vi "HEWH Water Cp.vi"(7 "Water Properties Reference":T1, 8 "Error In":errorcluster, 11 "Input Temperature (°F)":dbl format="%.4f") -> (0 "Error Out":errorcluster, 3 "Specific Heat (BTU/lbm*F)":dbl)   [LabVIEW 2019]
uses:
  Macros/UEF/Type Definitions/HEWH Water Properties.ctl
panel:
  out "Rounded Number":dbl
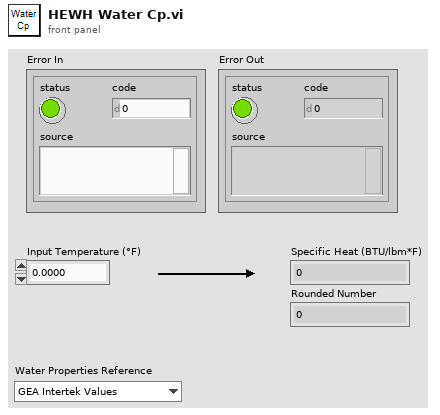
[diagram p1: front panel]
types:
  T1 = typedef "HEWH Water Properties.ctl" = enum16{"GEA Intertek Values", "CSA Values", "ANSI Values"}
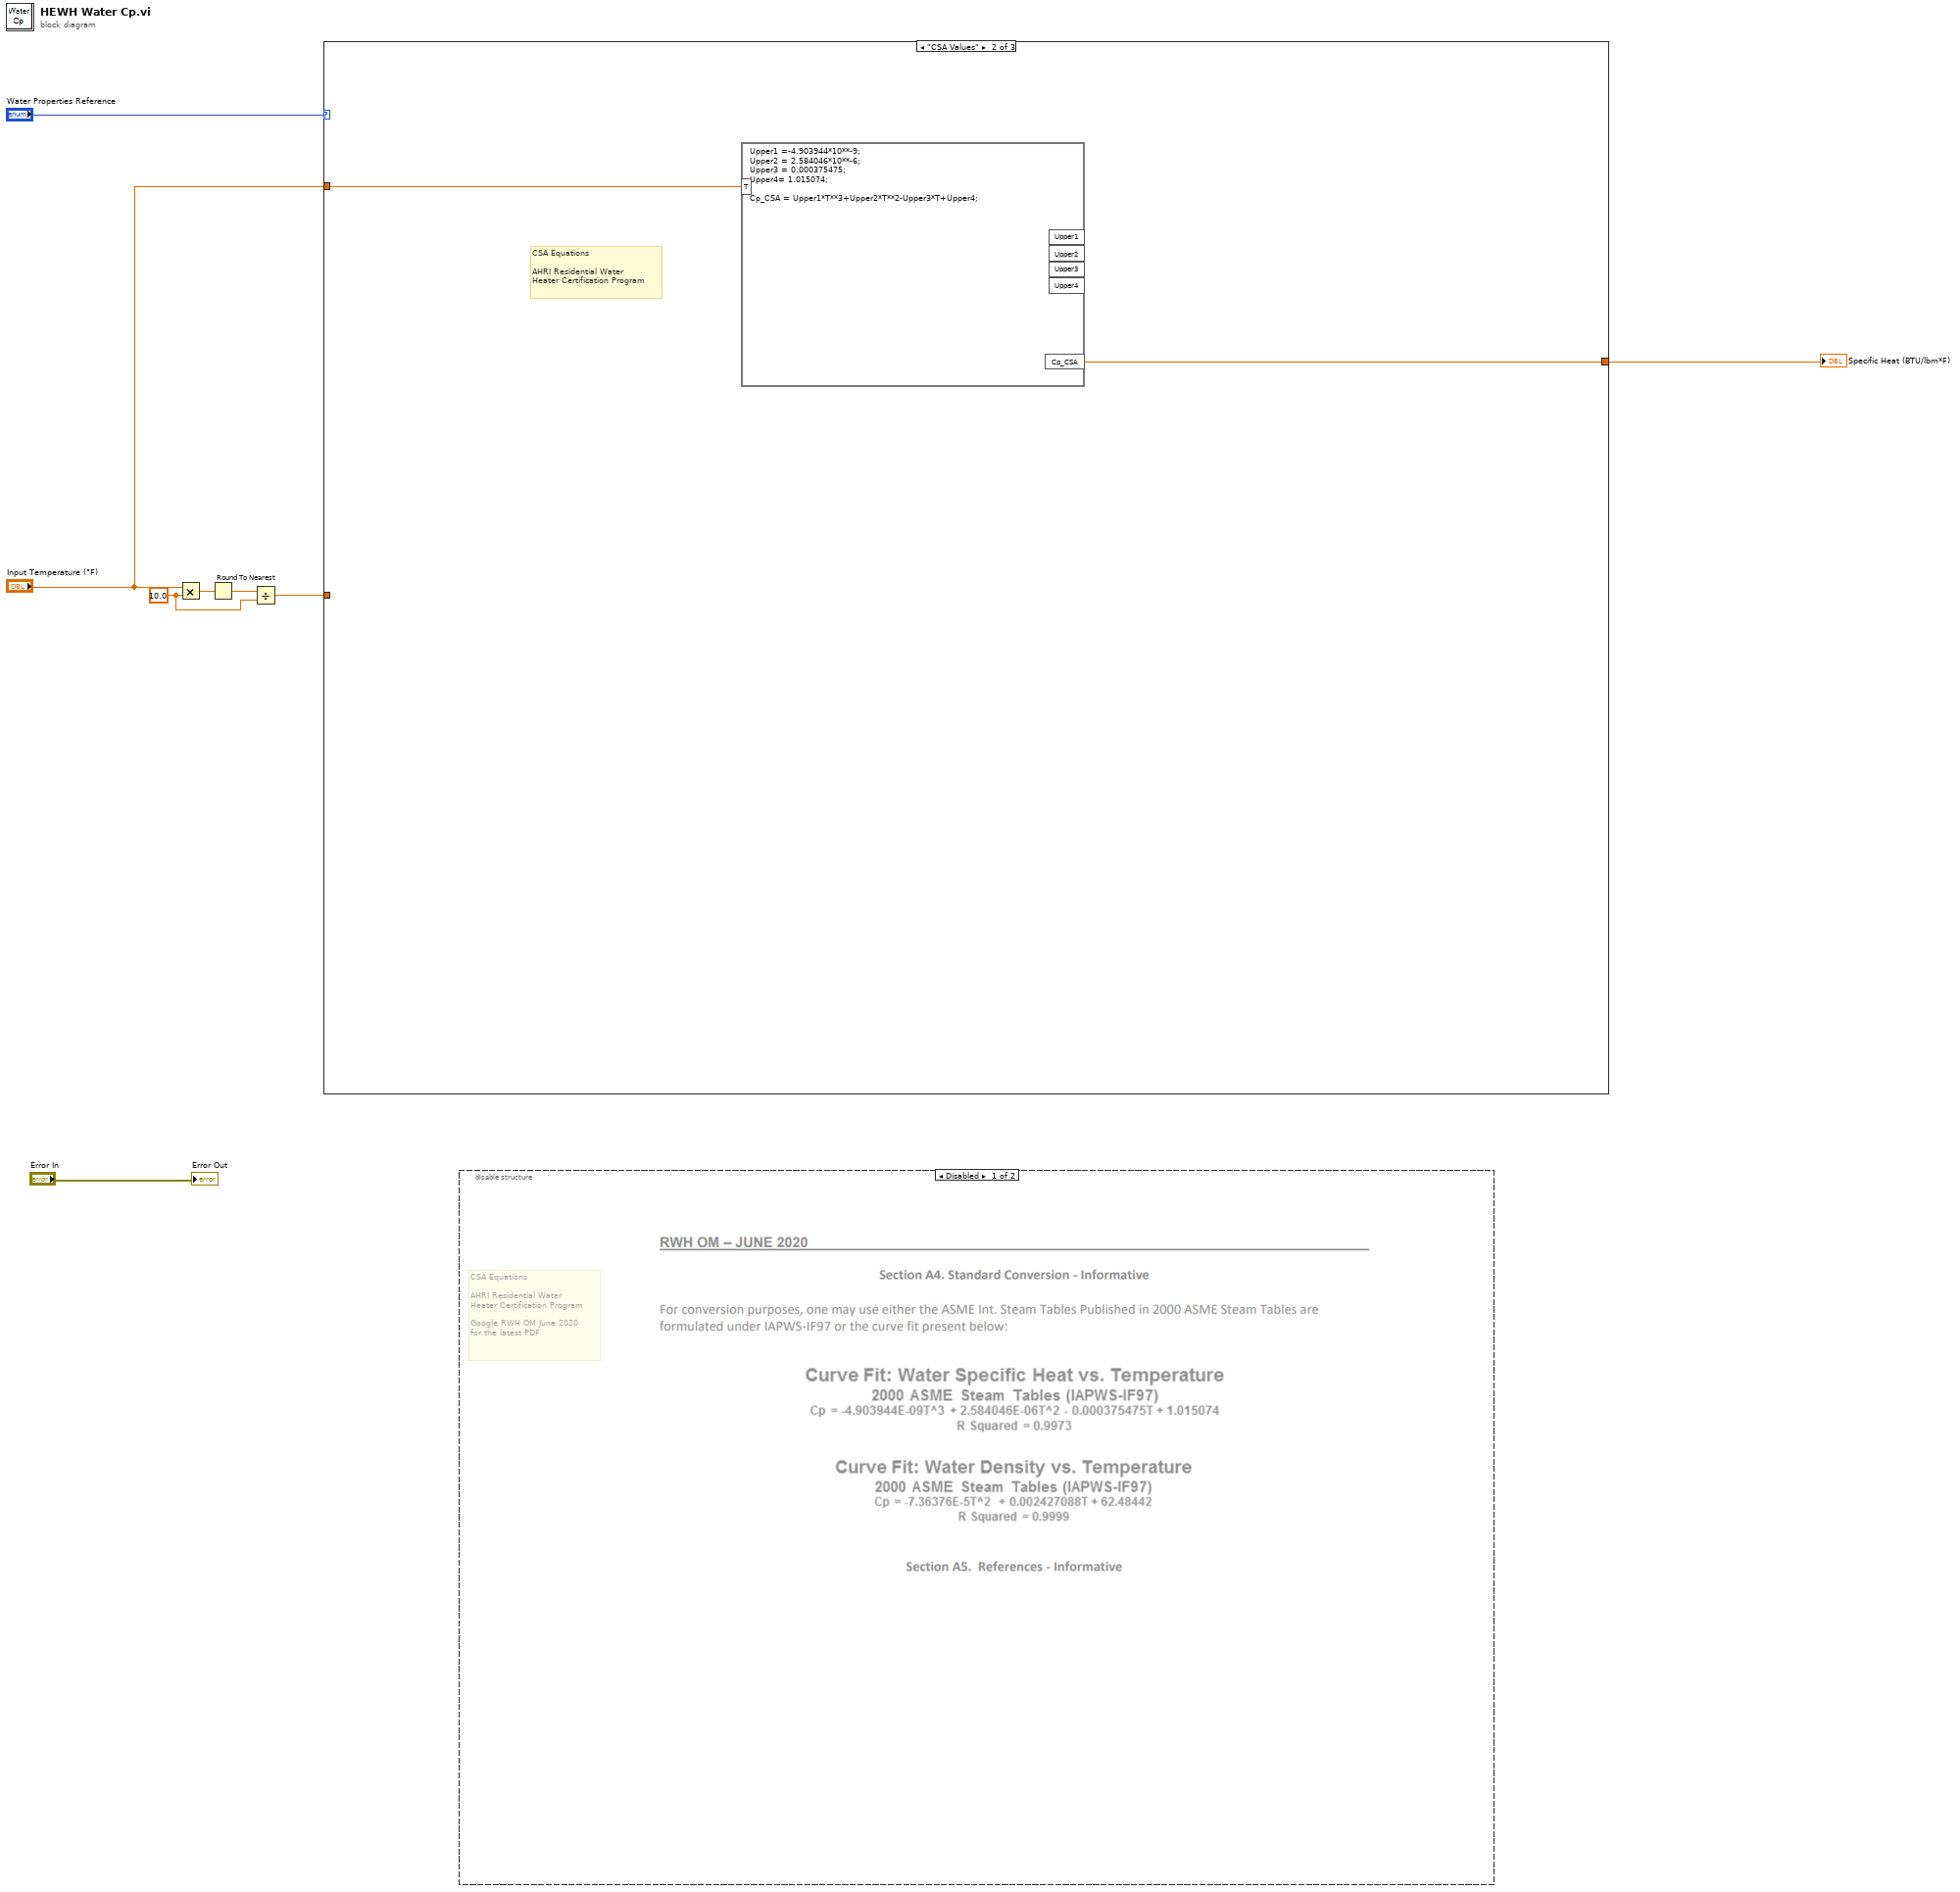
[diagram p0: block diagram]
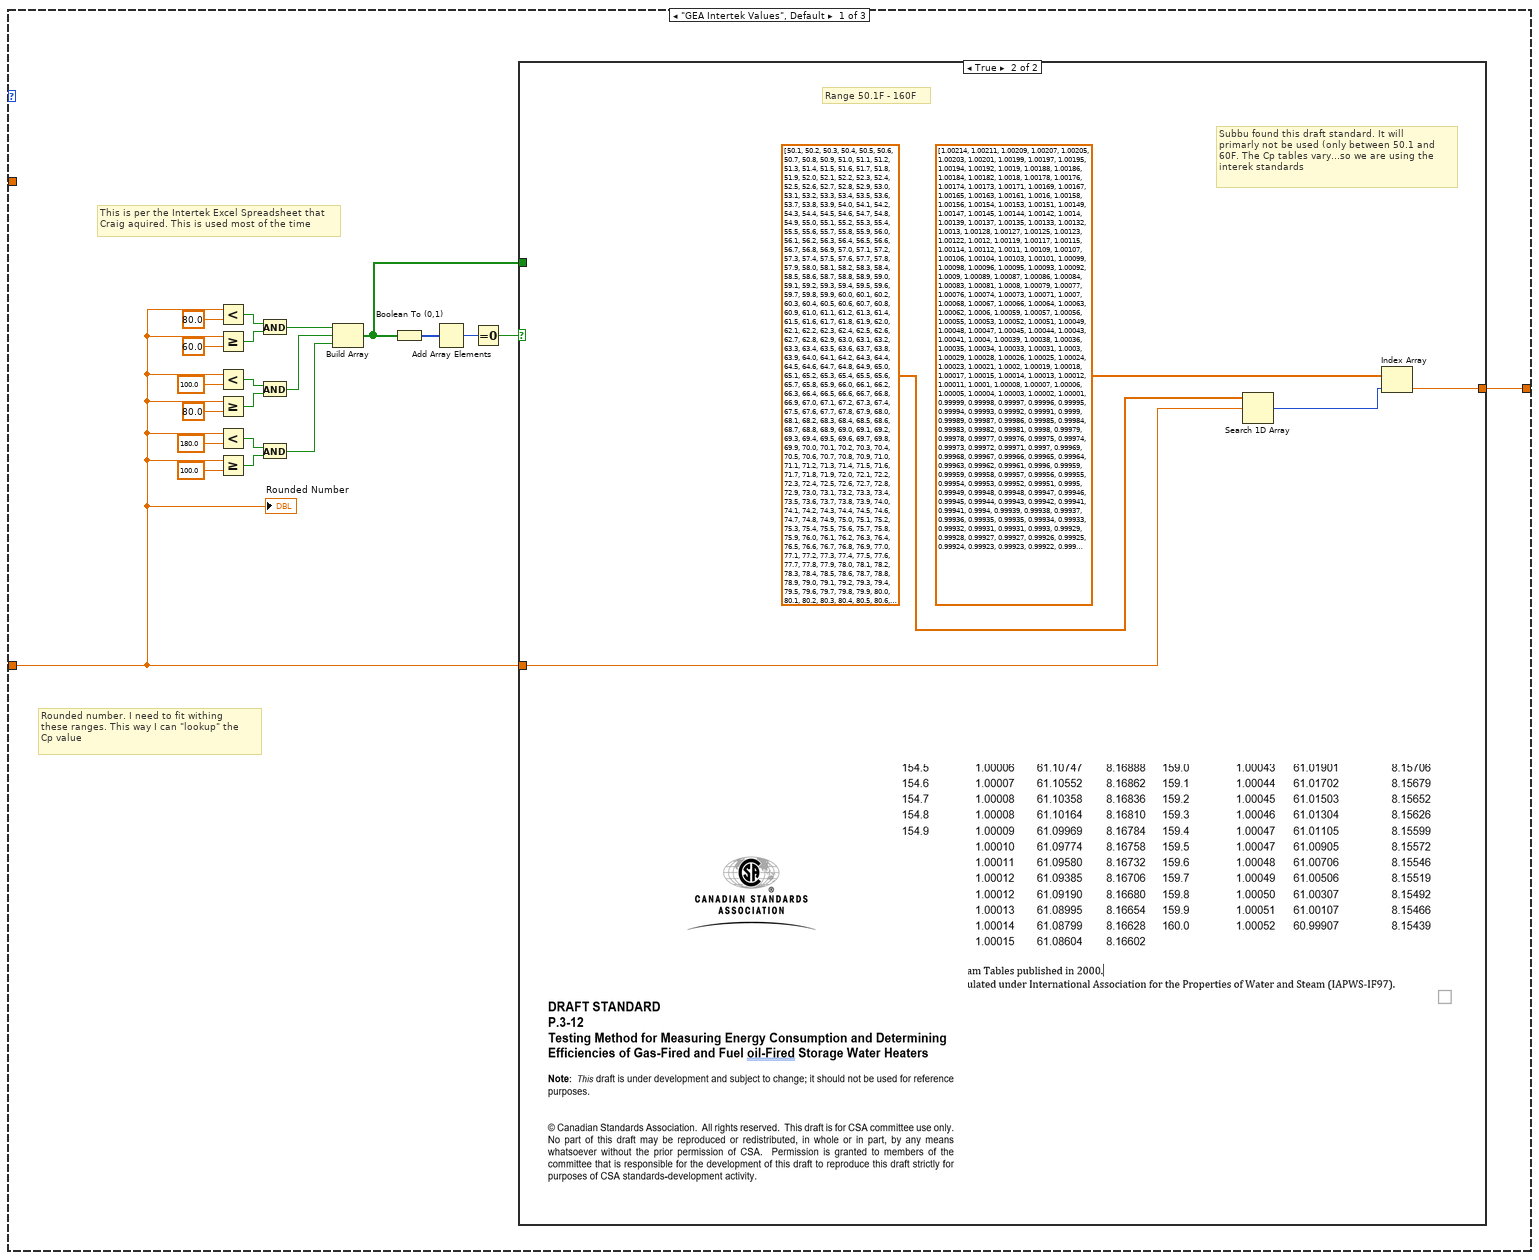
[diagram p3: hidden frame]
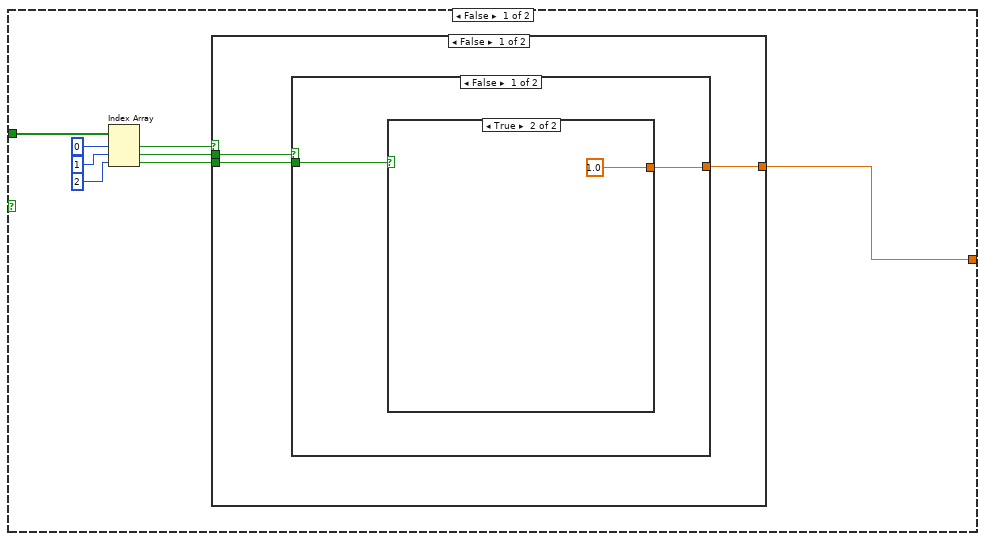
[diagram p4: hidden frame]
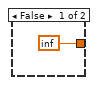
[diagram p5: hidden frame]
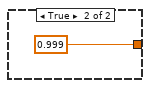
[diagram p6: hidden frame]
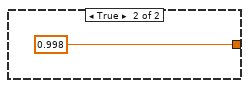
[diagram p7: hidden frame]
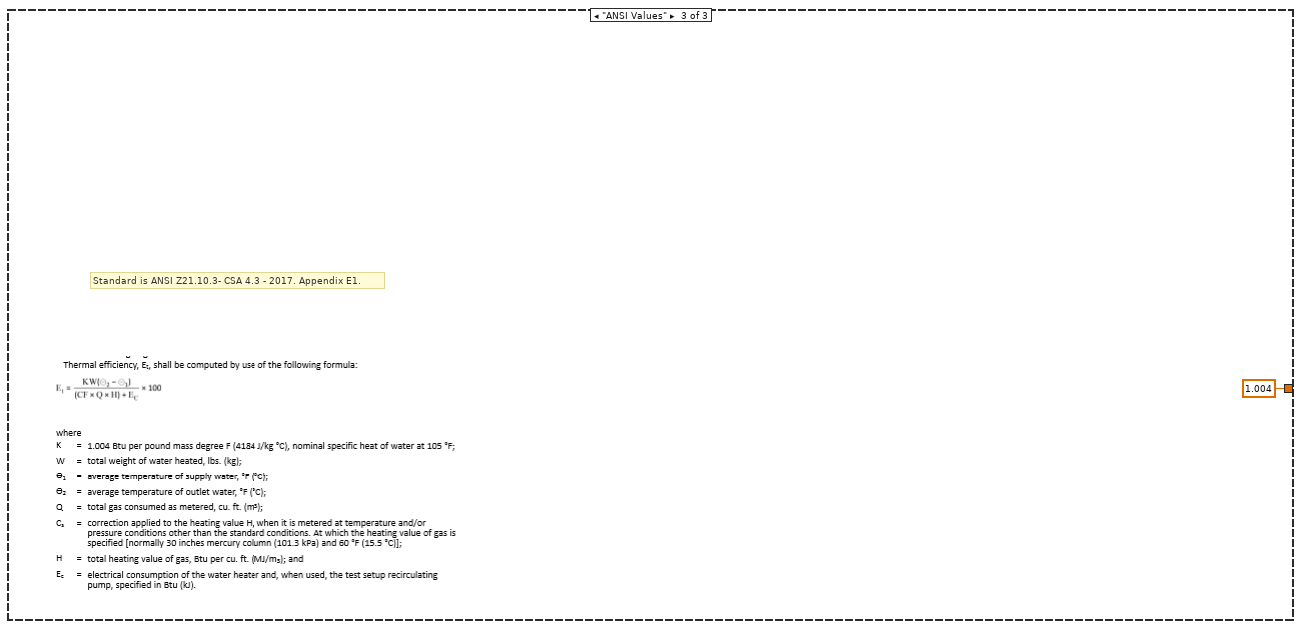
[diagram p8: hidden frame]
diagram:
  w4 = 10.0 ("y")
  n1 = Multiply(x="Input Temperature (°F)", y=w4) -> (x*y=w6:dbl)
  n2 = Round To Nearest(number=w6) -> (nearest integer value=w5:dbl)
  n3 = Divide(x=w5, y=w4) -> (x/y=w3:dbl)
  n4 = case shown="\"CSA Values\"" "Water Properties Reference" {
    tunnel: [w29 w52 1.004 ("Cp")] -> w7
    tunnel: w3 -> [w10 _ _]
    tunnel: "Input Temperature (°F)" -> [_ w53 _]
    frame "GEA Intertek Values", Default {
      # "Rounded number. I need to fit withing\nthese ranges. This way I can \"lookup\" the \nCp value"
      # "This is per the Intertek Excel Spreadsheet that \nCraig aquired. This is used most of the time"
      n5 = Less?(x=w10, y=80.0) -> (x < y?=w22:bool)
      n6 = Greater Or Equal?(x=w10, y=60.0) -> (x >= y?=w21:bool)
      n7 = Less?(x=w10, y=100.0) -> (x < y?=w20:bool)
      n8 = Greater Or Equal?(x=w10, y=80.0) -> (x >= y?=w19:bool)
      n9 = Less?(x=w10, y=180.0) -> (x < y?=w18:bool)
      n10 = Greater Or Equal?(x=w10, y=100.0) -> (x >= y?=w17:bool)
      n11 = And(x=w22, y=w21) -> (x .and. y?=w16:bool)
      n12 = And(x=w20, y=w19) -> (x .and. y?=w15:bool)
      n13 = And(x=w18, y=w17) -> (x .and. y?=w14:bool)
      n14 = Build Array(w16, w15, w14) -> (w11:bool[])
      n15 = Boolean To (0,1)(Boolean=w11) -> (0, 1=w13:i16[])
      n16 = Add Array Elements(numeric array=w13) -> (sum=w12:i16)
      n17 = Equal To 0?(x=w12) -> (x = 0?=w9:bool)
      n18 = case shown="True" w9 {
        tunnel: [w32 w47] -> w29
        tunnel: w10 -> [_ w51]
        tunnel: w11 -> [w37 _]
        frame False {
          n19 = Index Array(array=w37, index #1=0 ("index"), index #2=1 ("index"), index #3=2 ("index")) -> (element #1=w33:bool, element #2=w31:bool, element #3=w30:bool)
          n20 = case shown="False" w33 {
            tunnel: [w39 0.998 ("Cp")] -> w32
            tunnel: w31 -> [w40 _]
            tunnel: w30 -> [w38 _]
            frame False {
              n21 = case shown="False" w40 {
                tunnel: [w41 0.999 ("Cp")] -> w39
                tunnel: w38 -> [w42 _]
                frame False {
                  n22 = case shown="True" w42 {
                    tunnel: [inf 1.0 ("Cp")] -> w41
                    frame False {
                    }
                    frame True {
                    }
                  }
                }
                frame True {
                }
              }
            }
            frame True {
            }
          }
        }
        frame True {
          # "Subbu found this draft standard. It will\nprimarly not be used (only between 50.1 and \n60F. The Cp tables vary...so we are using the\ninterek standards"
          # "Range 50.1F - 160F"
          n23 = Search 1D Array(1D array=dbl[] [50.1, 50.2, 50.3, 50.4, 50.5, 50.6, 50.7, 50.8, 50.9, 51.0, 51.1, 51.2, 51.3, 51.4, 51.5, 51.6, 51.7, 51.8, 51.9, 52.0, 52.1, 52.2, 52.3, 52.4, 52.5, 52.6, 52.7, 52.8, 52.9, 53.0, 53.1, 53.2, 53.3, 53.4, 53.5, 53.6, 53.7, 53.8, 53.9, 54.0, 54.1, 54.2, 54.3, 54.4, 54.5, 54.6, 54.7, 54.8, 54.9, 55.0, 55.1, 55.2, 55.3, 55.4, 55.5, 55.6, 55.7, 55.8, 55.9, 56.0, 56.1, 56.2, 56.3, 56.4, 56.5, 56.6, 56.7, 56.8, 56.9, 57.0, 57.1, 57.2, 57.3, 57.4, 57.5, 57.6, 57.7, 57.8, 57.9, 58.0, 58.1, 58.2, 58.3, 58.4, 58.5, 58.6, 58.7, 58.8, 58.9, 59.0, 59.1, 59.2, 59.3, 59.4, 59.5, 59.6, 59.7, 59.8, 59.9, 60.0, 60.1, 60.2, 60.3, 60.4, 60.5, 60.6, 60.7, 60.8, 60.9, 61.0, 61.1, 61.2, 61.3, 61.4, 61.5, 61.6, 61.7, 61.8, 61.9, 62.0, 62.1, 62.2, 62.3, 62.4, 62.5, 62.6, 62.7, 62.8, 62.9, 63.0, 63.1, 63.2, 63.3, 63.4, 63.5, 63.6, 63.7, 63.8, 63.9, 64.0, 64.1, 64.2, 64.3, 64.4, 64.5, 64.6, 64.7, 64.8, 64.9, 65.0, 65.1, 65.2, 65.3, 65.4, 65.5, 65.6, 65.7, 65.8, 65.9, 66.0, 66.1, 66.2, 66.3, 66.4, 66.5, 66.6, 66.7, 66.8, 66.9, 67.0, 67.1, 67.2, 67.3, 67.4, 67.5, 67.6, 67.7, 67.8, 67.9, 68.0, 68.1, 68.2, 68.3, 68.4, 68.5, 68.6, 68.7, 68.8, 68.9, 69.0, 69.1, 69.2, 69.3, 69.4, 69.5, 69.6, 69.7, 69.8, 69.9, 70.0, 70.1, 70.2, 70.3, 70.4, 70.5, 70.6, 70.7, 70.8, 70.9, 71.0, 71.1, 71.2, 71.3, 71.4, 71.5, 71.6, 71.7, 71.8, 71.9, 72.0, 72.1, 72.2, 72.3, 72.4, 72.5, 72.6, 72.7, 72.8, 72.9, 73.0, 73.1, 73.2, 73.3, 73.4, 73.5, 73.6, 73.7, 73.8, 73.9, 74.0, 74.1, 74.2, 74.3, 74.4, 74.5, 74.6, 74.7, 74.8, 74.9, 75.0, 75.1, 75.2, 75.3, 75.4, 75.5, 75.6, 75.7, 75.8, 75.9, 76.0, 76.1, 76.2, 76.3, 76.4, 76.5, 76.6, 76.7, 76.8, 76.9, 77.0, 77.1, 77.2, 77.3, 77.4, 77.5, 77.6, 77.7, 77.8, 77.9, 78.0, 78.1, 78.2, 78.3, 78.4, 78.5, 78.6, 78.7, 78.8, 78.9, 79.0, 79.1, 79.2, 79.3, 79.4, 79.5, 79.6, 79.7, 79.8, 79.9, 80.0, 80.1, 80.2, 80.3, 80.4, 80.5, 80.6, 80.7, 80.8, 80.9, 81.0, 81.1, 81.2, 81.3, 81.4, 81.5, 81.6, 81.7, 81.8, 81.9, 82.0, 82.1, 82.2, 82.3, 82.4, 82.5, 82.6, 82.7, 82.8, 82.9, 83.0, 83.1, 83.2, 83.3, 83.4, 83.5, 83.6, 83.7, 83.8, 83.9, 84.0, 84.1, 84.2, 84.3, 84.4, 84.5, 84.6, 84.7, 84.8, 84.9, 85.0, 85.1, 85.2, 85.3, 85.4, 85.5, 85.6, 85.7, 85.8, 85.9, 86.0, 86.1, 86.2, 86.3, 86.4, 86.5, 86.6, 86.7, 86.8, 86.9, 87.0, 87.1, 87.2, 87.3, 87.4, 87.5, 87.6, 87.7, 87.8, 87.9, 88.0, 88.1, 88.2, 88.3, 88.4, 88.5, 88.6, 88.7, 88.8, 88.9, 89.0, 89.1, 89.2, 89.3, 89.4, 89.5, 89.6, 89.7, 89.8, 89.9, 90.0, 90.1, 90.2, 90.3, 90.4, 90.5, 90.6, 90.7, 90.8, 90.9, 91.0, 91.1, 91.2, 91.3, 91.4, 91.5, 91.6, 91.7, 91.8, 91.9, 92.0, 92.1, 92.2, 92.3, 92.4, 92.5, 92.6, 92.7, 92.8, 92.9, 93.0, 93.1, 93.2, 93.3, 93.4, 93.5, 93.6, 93.7, 93.8, 93.9, 94.0, 94.1, 94.2, 94.3, 94.4, 94.5, 94.6, 94.7, 94.8, 94.9, 95.0, 95.1, 95.2, 95.3, 95.4, 95.5, 95.6, 95.7, 95.8, 95.9, 96.0, 96.1, 96.2, 96.3, 96.4, 96.5, 96.6, 96.7, 96.8, 96.9, 97.0, 97.1, 97.2, 97.3, 97.4, 97.5, 97.6, 97.7, 97.8, 97.9, 98.0, 98.1, 98.2, 98.3, 98.4, 98.5, 98.6, 98.7, 98.8, 98.9, 99.0, 99.1, 99.2, 99.3, 99.4, 99.5, 99.6, 99.7, 99.8, 99.9, 100.0, 100.1, 100.2, 100.3, 100.4, 100.5, 100.6, 100.7, 100.8, 100.9, 101.0, 101.1, 101.2, 101.3, 101.4, 101.5, 101.6, 101.7, 101.8, 101.9, 102.0, 102.1, 102.2, 102.3, 102.4, 102.5, 102.6, 102.7, 102.8, 102.9, 103.0, 103.1, 103.2, 103.3, 103.4, 103.5, 103.6, 103.7, 103.8, 103.9, 104.0, 104.1, 104.2, 104.3, 104.4, 104.5, 104.6, 104.7, 104.8, 104.9, 105.0, 105.1, 105.2, 105.3, 105.4, 105.5, 105.6, 105.7, 105.8, 105.9, 106.0, 106.1, 106.2, 106.3, 106.4, 106.5, 106.6, 106.7, 106.8, 106.9, 107.0, 107.1, 107.2, 107.3, 107.4, 107.5, 107.6, 107.7, 107.8, 107.9, 108.0, 108.1, 108.2, 108.3, 108.4, 108.5, 108.6, 108.7, 108.8, 108.9, 109.0, 109.1, 109.2, 109.3, 109.4, 109.5, 109.6, 109.7, 109.8, 109.9, 110.0, 110.1, 110.2, 110.3, 110.4, 110.5, 110.6, 110.7, 110.8, 110.9, 111.0, 111.1, 111.2, 111.3, 111.4, 111.5, 111.6, 111.7, 111.8, 111.9, 112.0, 112.1, 112.2, 112.3, 112.4, 112.5, 112.6, 112.7, 112.8, 112.9, 113.0, 113.1, 113.2, 113.3, 113.4, 113.5, 113.6, 113.7, 113.8, 113.9, 114.0, 114.1, 114.2, 114.3, 114.4, 114.5, 114.6, 114.7, 114.8, 114.9, 115.0, 115.1, 115.2, 115.3, 115.4, 115.5, 115.6, 115.7, 115.8, 115.9, 116.0, 116.1, 116.2, 116.3, 116.4, 116.5, 116.6, 116.7, 116.8, 116.9, 117.0, 117.1, 117.2, 117.3, 117.4, 117.5, 117.6, 117.7, 117.8, 117.9, 118.0, 118.1, 118.2, 118.3, 118.4, 118.5, 118.6, 118.7, 118.8, 118.9, 119.0, 119.1, 119.2, 119.3, 119.4, 119.5, 119.6, 119.7, 119.8, 119.9, 120.0, 120.1, 120.2, 120.3, 120.4, 120.5, 120.6, 120.7, 120.8, 120.9, 121.0, 121.1, 121.2, 121.3, 121.4, 121.5, 121.6, 121.7, 121.8, 121.9, 122.0, 122.1, 122.2, 122.3, 122.4, 122.5, 122.6, 122.7, 122.8, 122.9, 123.0, 123.1, 123.2, 123.3, 123.4, 123.5, 123.6, 123.7, 123.8, 123.9, 124.0, 124.1, 124.2, 124.3, 124.4, 124.5, 124.6, 124.7, 124.8, 124.9, 125.0, 125.1, 125.2, 125.3, 125.4, 125.5, 125.6, 125.7, 125.8, 125.9, 126.0, 126.1, 126.2, 126.3, 126.4, 126.5, 126.6, 126.7, 126.8, 126.9, 127.0, 127.1, 127.2, 127.3, 127.4, 127.5, 127.6, 127.7, 127.8, 127.9, 128.0, 128.1, 128.2, 128.3, 128.4, 128.5, 128.6, 128.7, 128.8, 128.9, 129.0, 129.1, 129.2, 129.3, 129.4, 129.5, 129.6, 129.7, 129.8, 129.9, 130.0, 130.1, 130.2, 130.3, 130.4, 130.5, 130.6, 130.7, 130.8, 130.9, 131.0, 131.1, 131.2, 131.3, 131.4, 131.5, 131.6, 131.7, 131.8, 131.9, 132.0, 132.1, 132.2, 132.3, 132.4, 132.5, 132.6, 132.7, 132.8, 132.9, 133.0, 133.1, 133.2, 133.3, 133.4, 133.5, 133.6, 133.7, 133.8, 133.9, 134.0, 134.1, 134.2, 134.3, 134.4, 134.5, 134.6, 134.7, 134.8, 134.9, 135.0, 135.1, 135.2, 135.3, 135.4, 135.5, 135.6, 135.7, 135.8, 135.9, 136.0, 136.1, 136.2, 136.3, 136.4, 136.5, 136.6, 136.7, 136.8, 136.9, 137.0, 137.1, 137.2, 137.3, 137.4, 137.5, 137.6, 137.7, 137.8, 137.9, 138.0, 138.1, 138.2, 138.3, 138.4, 138.5, 138.6, 138.7, 138.8, 138.9, 139.0, 139.1, 139.2, 139.3, 139.4, 139.5, 139.6, 139.7, 139.8, 139.9, 140.0, 140.1, 140.2, 140.3, 140.4, 140.5, 140.6, 140.7, 140.8, 140.9, 141.0, 141.1, 141.2, 141.3, 141.4, 141.5, 141.6, 141.7, 141.8, 141.9, 142.0, 142.1, 142.2, 142.3, 142.4, 142.5, 142.6, 142.7, 142.8, 142.9, 143.0, 143.1, 143.2, 143.3, 143.4, 143.5, 143.6, 143.7, 143.8, 143.9, 144.0, 144.1, 144.2, 144.3, 144.4, 144.5, 144.6, 144.7, 144.8, 144.9, 145.0, 145.1, 145.2, 145.3, 145.4, 145.5, 145.6, 145.7, 145.8, 145.9, 146.0, 146.1, 146.2, 146.3, 146.4, 146.5, 146.6, 146.7, 146.8, 146.9, 147.0, 147.1, 147.2, 147.3, 147.4, 147.5, 147.6, 147.7, 147.8, 147.9, 148.0, 148.1, 148.2, 148.3, 148.4, 148.5, 148.6, 148.7, 148.8, 148.9, 149.0, 149.1, 149.2, 149.3, 149.4, 149.5, 149.6, 149.7, 149.8, 149.9, 150.0, 150.1, 150.2, 150.3, 150.4, 150.5, 150.6, 150.7, 150.8, 150.9, 151.0, 151.1, 151.2, 151.3, 151.4, 151.5, 151.6, 151.7, 151.8, 151.9, 152.0, 152.1, 152.2, 152.3, 152.4, 152.5, 152.6, 152.7, 152.8, 152.9, 153.0, 153.1, 153.2, 153.3, 153.4, 153.5, 153.6, 153.7, 153.8, 153.9, 154.0, 154.1, 154.2, 154.3, 154.4, 154.5, 154.6, 154.7, 154.8, 154.9, 155.0, 155.1, 155.2, 155.3, 155.4, 155.5, 155.6, 155.7, 155.8, 155.9, 156.0, 156.1, 156.2, 156.3, 156.4, 156.5, 156.6, 156.7, 156.8, 156.9, 157.0, 157.1, 157.2, 157.3, 157.4, 157.5, 157.6, 157.7, 157.8, 157.9, 158.0, 158.1, 158.2, 158.3, 158.4, 158.5, 158.6, 158.7, 158.8, 158.9, 159.0, 159.1, 159.2, 159.3, 159.4, 159.5, 159.6, 159.7, 159.8, 159.9, 160.0] ("Array"), element=w51) -> (index of element=w48:i32)  [unwired: 1 in]
          n24 = Index Array(array=dbl[] [1.00214, 1.00211, 1.00209, 1.00207, 1.00205, 1.00203, 1.00201, 1.00199, 1.00197, 1.00195, 1.00194, 1.00192, 1.0019, 1.00188, 1.00186, 1.00184, 1.00182, 1.0018, 1.00178, 1.00176, 1.00174, 1.00173, 1.00171, 1.00169, 1.00167, 1.00165, 1.00163, 1.00161, 1.0016, 1.00158, 1.00156, 1.00154, 1.00153, 1.00151, 1.00149, 1.00147, 1.00145, 1.00144, 1.00142, 1.0014, 1.00139, 1.00137, 1.00135, 1.00133, 1.00132, 1.0013, 1.00128, 1.00127, 1.00125, 1.00123, 1.00122, 1.0012, 1.00119, 1.00117, 1.00115, 1.00114, 1.00112, 1.0011, 1.00109, 1.00107, 1.00106, 1.00104, 1.00103, 1.00101, 1.00099, 1.00098, 1.00096, 1.00095, 1.00093, 1.00092, 1.0009, 1.00089, 1.00087, 1.00086, 1.00084, 1.00083, 1.00081, 1.0008, 1.00079, 1.00077, 1.00076, 1.00074, 1.00073, 1.00071, 1.0007, 1.00068, 1.00067, 1.00066, 1.00064, 1.00063, 1.00062, 1.0006, 1.00059, 1.00057, 1.00056, 1.00055, 1.00053, 1.00052, 1.00051, 1.00049, 1.00048, 1.00047, 1.00045, 1.00044, 1.00043, 1.00041, 1.0004, 1.00039, 1.00038, 1.00036, 1.00035, 1.00034, 1.00033, 1.00031, 1.0003, 1.00029, 1.00028, 1.00026, 1.00025, 1.00024, 1.00023, 1.00021, 1.0002, 1.00019, 1.00018, 1.00017, 1.00015, 1.00014, 1.00013, 1.00012, 1.00011, 1.0001, 1.00008, 1.00007, 1.00006, 1.00005, 1.00004, 1.00003, 1.00002, 1.00001, 0.99999, 0.99998, 0.99997, 0.99996, 0.99995, 0.99994, 0.99993, 0.99992, 0.99991, 0.9999, 0.99989, 0.99987, 0.99986, 0.99985, 0.99984, 0.99983, 0.99982, 0.99981, 0.9998, 0.99979, 0.99978, 0.99977, 0.99976, 0.99975, 0.99974, 0.99973, 0.99972, 0.99971, 0.9997, 0.99969, 0.99968, 0.99967, 0.99966, 0.99965, 0.99964, 0.99963, 0.99962, 0.99961, 0.9996, 0.99959, 0.99959, 0.99958, 0.99957, 0.99956, 0.99955, 0.99954, 0.99953, 0.99952, 0.99951, 0.9995, 0.99949, 0.99948, 0.99948, 0.99947, 0.99946, 0.99945, 0.99944, 0.99943, 0.99942, 0.99941, 0.99941, 0.9994, 0.99939, 0.99938, 0.99937, 0.99936, 0.99935, 0.99935, 0.99934, 0.99933, 0.99932, 0.99931, 0.99931, 0.9993, 0.99929, 0.99928, 0.99927, 0.99927, 0.99926, 0.99925, 0.99924, 0.99923, 0.99923, 0.99922, 0.99921, 0.9992, 0.99919, 0.99919, 0.99918, 0.99917, 0.99916, 0.99916, 0.99915, 0.99914, 0.99913, 0.99913, 0.99912, 0.99911, 0.99911, 0.9991, 0.99909, 0.99908, 0.99908, 0.99907, 0.99906, 0.99906, 0.99905, 0.99904, 0.99903, 0.99903, 0.99902, 0.99901, 0.99901, 0.999, 0.99899, 0.99899, 0.99898, 0.99897, 0.99897, 0.99896, 0.99895, 0.99895, 0.99894, 0.99893, 0.99893, 0.99892, 0.99892, 0.99891, 0.9989, 0.9989, 0.99889, 0.99888, 0.99888, 0.99887, 0.99887, 0.99886, 0.99885, 0.99885, 0.99884, 0.99884, 0.99883, 0.99882, 0.99882, 0.99881, 0.99881, 0.9988, 0.99879, 0.99879, 0.99878, 0.99878, 0.99877, 0.99877, 0.99876, 0.99875, 0.99875, 0.99874, 0.99874, 0.99873, 0.99873, 0.99872, 0.99872, 0.99871, 0.99871, 0.9987, 0.99869, 0.99869, 0.99868, 0.99868, 0.99867, 0.99867, 0.99866, 0.99866, 0.99865, 0.99865, 0.99864, 0.99864, 0.99863, 0.99863, 0.99862, 0.99862, 0.99861, 0.99861, 0.9986, 0.9986, 0.99859, 0.99859, 0.99859, 0.99858, 0.99858, 0.99857, 0.99857, 0.99856, 0.99856, 0.99855, 0.99855, 0.99854, 0.99854, 0.99853, 0.99853, 0.99853, 0.99852, 0.99852, 0.99851, 0.99851, 0.9985, 0.9985, 0.9985, 0.99849, 0.99849, 0.99848, 0.99848, 0.99848, 0.99847, 0.99847, 0.99846, 0.99846, 0.99846, 0.99845, 0.99845, 0.99844, 0.99844, 0.99844, 0.99843, 0.99843, 0.99842, 0.99842, 0.99842, 0.99841, 0.99841, 0.99841, 0.9984, 0.9984, 0.99839, 0.99839, 0.99839, 0.99838, 0.99838, 0.99838, 0.99837, 0.99837, 0.99837, 0.99836, 0.99836, 0.99836, 0.99835, 0.99835, 0.99835, 0.99834, 0.99834, 0.99834, 0.99833, 0.99833, 0.99833, 0.99832, 0.99832, 0.99832, 0.99832, 0.99831, 0.99831, 0.99831, 0.9983, 0.9983, 0.9983, 0.99829, 0.99829, 0.99829, 0.99829, 0.99828, 0.99828, 0.99828, 0.99827, 0.99827, 0.99827, 0.99827, 0.99826, 0.99826, 0.99826, 0.99826, 0.99825, 0.99825, 0.99825, 0.99825, 0.99824, 0.99824, 0.99824, 0.99824, 0.99823, 0.99823, 0.99823, 0.99823, 0.99822, 0.99822, 0.99822, 0.99822, 0.99821, 0.99821, 0.99821, 0.99821, 0.99821, 0.9982, 0.9982, 0.9982, 0.9982, 0.9982, 0.99819, 0.99819, 0.99819, 0.99819, 0.99819, 0.99818, 0.99818, 0.99818, 0.99818, 0.99818, 0.99817, 0.99817, 0.99817, 0.99817, 0.99817, 0.99816, 0.99816, 0.99816, 0.99816, 0.99816, 0.99816, 0.99815, 0.99815, 0.99815, 0.99815, 0.99815, 0.99815, 0.99815, 0.99814, 0.99814, 0.99814, 0.99814, 0.99814, 0.99814, 0.99813, 0.99813, 0.99813, 0.99813, 0.99813, 0.99813, 0.99813, 0.99813, 0.99812, 0.99812, 0.99812, 0.99812, 0.99812, 0.99812, 0.99812, 0.99812, 0.99812, 0.99811, 0.99811, 0.99811, 0.99811, 0.99811, 0.99811, 0.99811, 0.99811, 0.99811, 0.99811, 0.9981, 0.9981, 0.9981, 0.9981, 0.9981, 0.9981, 0.9981, 0.9981, 0.9981, 0.9981, 0.9981, 0.9981, 0.9981, 0.99809, 0.99809, 0.99809, 0.99809, 0.99809, 0.99809, 0.99809, 0.99809, 0.99809, 0.99809, 0.99809, 0.99809, 0.99809, 0.99809, 0.99809, 0.99809, 0.99809, 0.99809, 0.99809, 0.99809, 0.99809, 0.99809, 0.99809, 0.99809, 0.99808, 0.99808, 0.99808, 0.99808, 0.99808, 0.99808, 0.99808, 0.99808, 0.99808, 0.99808, 0.99808, 0.99808, 0.99808, 0.99808, 0.99808, 0.99808, 0.99808, 0.99808, 0.99808, 0.99808, 0.99808, 0.99808, 0.99808, 0.99808, 0.99809, 0.99809, 0.99809, 0.99809, 0.99809, 0.99809, 0.99809, 0.99809, 0.99809, 0.99809, 0.99809, 0.99809, 0.99809, 0.99809, 0.99809, 0.99809, 0.99809, 0.99809, 0.99809, 0.99809, 0.99809, 0.99809, 0.99809, 0.99809, 0.9981, 0.9981, 0.9981, 0.9981, 0.9981, 0.9981, 0.9981, 0.9981, 0.9981, 0.9981, 0.9981, 0.9981, 0.9981, 0.99811, 0.99811, 0.99811, 0.99811, 0.99811, 0.99811, 0.99811, 0.99811, 0.99811, 0.99811, 0.99811, 0.99812, 0.99812, 0.99812, 0.99812, 0.99812, 0.99812, 0.99812, 0.99812, 0.99812, 0.99813, 0.99813, 0.99813, 0.99813, 0.99813, 0.99813, 0.99813, 0.99814, 0.99814, 0.99814, 0.99814, 0.99814, 0.99814, 0.99814, 0.99814, 0.99815, 0.99815, 0.99815, 0.99815, 0.99815, 0.99815, 0.99816, 0.99816, 0.99816, 0.99816, 0.99816, 0.99816, 0.99816, 0.99817, 0.99817, 0.99817, 0.99817, 0.99817, 0.99818, 0.99818, 0.99818, 0.99818, 0.99818, 0.99818, 0.99819, 0.99819, 0.99819, 0.99819, 0.99819, 0.9982, 0.9982, 0.9982, 0.9982, 0.9982, 0.99821, 0.99821, 0.99821, 0.99821, 0.99821, 0.99822, 0.99822, 0.99822, 0.99822, 0.99822, 0.99823, 0.99823, 0.99823, 0.99823, 0.99824, 0.99824, 0.99824, 0.99824, 0.99824, 0.99825, 0.99825, 0.99825, 0.99825, 0.99826, 0.99826, 0.99826, 0.99826, 0.99827, 0.99827, 0.99827, 0.99827, 0.99828, 0.99828, 0.99828, 0.99828, 0.99829, 0.99829, 0.99829, 0.99829, 0.9983, 0.9983, 0.9983, 0.9983, 0.99831, 0.99831, 0.99831, 0.99832, 0.99832, 0.99832, 0.99832, 0.99833, 0.99833, 0.99833, 0.99834, 0.99834, 0.99834, 0.99834, 0.99835, 0.99835, 0.99835, 0.99836, 0.99836, 0.99836, 0.99837, 0.99837, 0.99837, 0.99837, 0.99838, 0.99838, 0.99838, 0.99839, 0.99839, 0.99839, 0.9984, 0.9984, 0.9984, 0.99841, 0.99841, 0.99841, 0.99842, 0.99842, 0.99842, 0.99843, 0.99843, 0.99843, 0.99844, 0.99844, 0.99844, 0.99845, 0.99845, 0.99845, 0.99846, 0.99846, 0.99846, 0.99847, 0.99847, 0.99847, 0.99848, 0.99848, 0.99849, 0.99849, 0.99849, 0.9985, 0.9985, 0.9985, 0.99851, 0.99851, 0.99851, 0.99852, 0.99852, 0.99853, 0.99853, 0.99853, 0.99854, 0.99854, 0.99855, 0.99855, 0.99855, 0.99856, 0.99856, 0.99857, 0.99857, 0.99857, 0.99858, 0.99858, 0.99859, 0.99859, 0.99859, 0.9986, 0.9986, 0.99861, 0.99861, 0.99861, 0.99862, 0.99862, 0.99863, 0.99863, 0.99863, 0.99864, 0.99864, 0.99865, 0.99865, 0.99866, 0.99866, 0.99866, 0.99867, 0.99867, 0.99868, 0.99868, 0.99869, 0.99869, 0.9987, 0.9987, 0.9987, 0.99871, 0.99871, 0.99872, 0.99872, 0.99873, 0.99873, 0.99874, 0.99874, 0.99875, 0.99875, 0.99875, 0.99876, 0.99876, 0.99877, 0.99877, 0.99878, 0.99878, 0.99879, 0.99879, 0.9988, 0.9988, 0.99881, 0.99881, 0.99882, 0.99882, 0.99883, 0.99883, 0.99884, 0.99884, 0.99885, 0.99885, 0.99886, 0.99886, 0.99887, 0.99887, 0.99888, 0.99888, 0.99889, 0.99889, 0.9989, 0.9989, 0.99891, 0.99891, 0.99892, 0.99892, 0.99893, 0.99893, 0.99894, 0.99894, 0.99895, 0.99895, 0.99896, 0.99896, 0.99897, 0.99897, 0.99898, 0.99899, 0.99899, 0.999, 0.999, 0.99901, 0.99901, 0.99902, 0.99902, 0.99903, 0.99903, 0.99904, 0.99905, 0.99905, 0.99906, 0.99906, 0.99907, 0.99907, 0.99908, 0.99908, 0.99909, 0.9991, 0.9991, 0.99911, 0.99911, 0.99912, 0.99912, 0.99913, 0.99914, 0.99914, 0.99915, 0.99915, 0.99916, 0.99917, 0.99917, 0.99918, 0.99918, 0.99919, 0.9992, 0.9992, 0.99921, 0.99921, 0.99922, 0.99923, 0.99923, 0.99924, 0.99924, 0.99925, 0.99926, 0.99926, 0.99927, 0.99927, 0.99928, 0.99929, 0.99929, 0.9993, 0.9993, 0.99931, 0.99932, 0.99932, 0.99933, 0.99934, 0.99934, 0.99935, 0.99936, 0.99936, 0.99937, 0.99937, 0.99938, 0.99939, 0.99939, 0.9994, 0.99941, 0.99941, 0.99942, 0.99943, 0.99943, 0.99944, 0.99945, 0.99945, 0.99946, 0.99947, 0.99947, 0.99948, 0.99949, 0.99949, 0.9995, 0.99951, 0.99951, 0.99952, 0.99953, 0.99953, 0.99954, 0.99955, 0.99955, 0.99956, 0.99957, 0.99957, 0.99958, 0.99959, 0.99959, 0.9996, 0.99961, 0.99962, 0.99962, 0.99963, 0.99964, 0.99964, 0.99965, 0.99966, 0.99966, 0.99967, 0.99968, 0.99969, 0.99969, 0.9997, 0.99971, 0.99971, 0.99972, 0.99973, 0.99974, 0.99974, 0.99975, 0.99976, 0.99976, 0.99977, 0.99978, 0.99979, 0.99979, 0.9998, 0.99981, 0.99982, 0.99982, 0.99983, 0.99984, 0.99985, 0.99985, 0.99986, 0.99987, 0.99988, 0.99988, 0.99989, 0.9999, 0.99991, 0.99991, 0.99992, 0.99993, 0.99994, 0.99994, 0.99995, 0.99996, 0.99997, 0.99997, 0.99998, 0.99999, 1.0, 1.00001, 1.00001, 1.00002, 1.00003, 1.00004, 1.00004, 1.00005, 1.00006, 1.00007, 1.00008, 1.00008, 1.00009, 1.0001, 1.00011, 1.00012, 1.00012, 1.00013, 1.00014, 1.00015, 1.00016, 1.00016, 1.00017, 1.00018, 1.00019, 1.0002, 1.00021, 1.00021, 1.00022, 1.00023, 1.00024, 1.00025, 1.00025, 1.00026, 1.00027, 1.00028, 1.00029, 1.0003, 1.0003, 1.00031, 1.00032, 1.00033, 1.00034, 1.00035, 1.00035, 1.00036, 1.00037, 1.00038, 1.00039, 1.0004, 1.00041, 1.00041, 1.00042, 1.00043, 1.00044, 1.00045, 1.00046, 1.00047, 1.00047, 1.00048, 1.00049, 1.0005, 1.00051, 1.00052] ("Array 2"), index=w48) -> (element=w47:dbl)
        }
      }
      "Rounded Number" <- w10
    }
    frame "CSA Values" {
      # "CSA Equations\n\nAHRI Residential Water\nHeater Certification Program"
      n25 = formula code="Upper1 =-4.903944*10**-9; \nUpper2 = 2.584046*10**-6;\nUpper3 = 0.000375475;\nUpper4= 1.015074;\n\nCp_CSA = Upper1*T**3+Upper2*T**2-Upper3*T+Upper4;"("T"=w53) -> ("Cp_CSA"=w52:dbl)  [unwired: 4 out]
    }
    frame "ANSI Values" {
      # "Standard is ANSI Z21.10.3- CSA 4.3 - 2017. Appendix E1."
    }
  }
  "Specific Heat (BTU/lbm*F)" <- w7
  n26 = disable-structure shown="Disabled" {
    frame Disabled {
      # "CSA Equations\n\nAHRI Residential Water\nHeater Certification Program\n\nGoogle RWH OM June 2020\nfor the latest PDF"
    }
    frame Enabled {
    }
  }
  "Error Out" <- "Error In"
